vi "Inverse Square Root 2.vi"() -> ()   [LabVIEW 2022 SP3, in "3D.lvlib"]
uses:
  3ca7c682-72f9-471a-94d6-f3f625e42330.vi
  717569c3-c8f8-4444-b08c-2f89a2934aa8.vi
  <vilib>/Utility/High Resolution Relative Seconds.vi
  3D.lvlib
  <vilib>/Analysis/NI_AALBase.lvlib
panel:
  out "Std Dev":dbl format="%.1p"
  out "Mean":dbl format="%.1p"
  out "Histogram Graph":T1(graph)
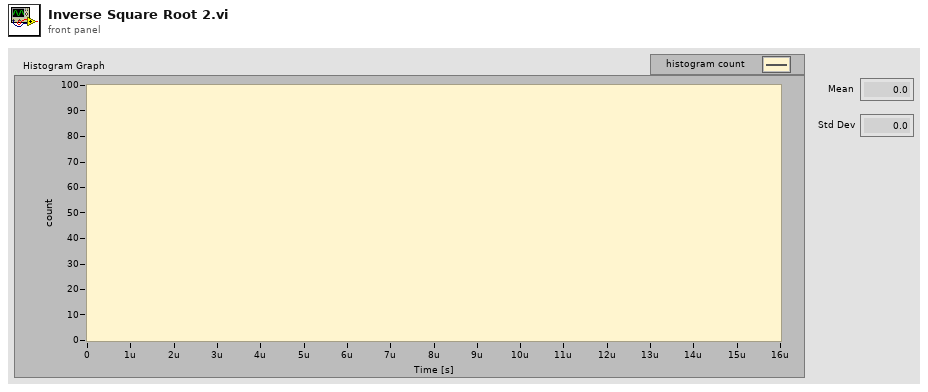
[diagram p1: front panel]
types:
  T1 = cluster{"X Values":dbl[], "Histogram: h(x)":i32[]}
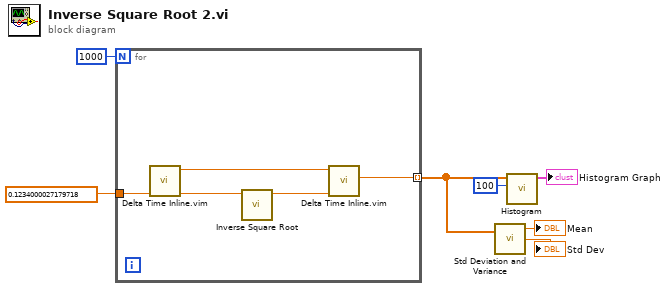
[diagram p0: block diagram]
diagram:
  n1 = for {
    N: 1000 -> [_]
    tunnel: [w12] -> w4 mode=indexing
    tunnel: sgl 0.1234 -> [w10]
    n2 = call "Delta Time Inline.vim"("value in"=w10) -> ("value out"=w9:sgl, "Relative Seconds out [s]"=w11:dbl)  [unwired: 8 in, 1 out]
    n3 = call "Inverse Square Root.vi"("Numeric"=w9) -> ("Inverse Square Root"=w8:sgl)  [unwired: 10 in]
    n4 = call "Delta Time Inline.vim"("value in"=w8, "Relative Seconds in [s]"=w11) -> ("Delta Time [s]"=w12:dbl)  [unwired: 7 in, 2 out]
  }
  n5 = call <vilib>:"Std Deviation and Variance.vi"("X"=w4) -> ("mean"=→"Mean":dbl, "standard deviation"=→"Std Dev":dbl)  [unwired: 1 in, 1 out]
  n6 = call <vilib>:"Histogram.vi"("intervals"=100, "X"=w4) -> ("Histogram Graph"=→"Histogram Graph":T1)  [unwired: 6 in, 3 out]
